vi "URL Equipos.vi"() -> ()   [LabVIEW 2018]
uses:
  <vilib>/RAFA Solutions/Harmony UI Controls Kit/Boolean/Blank Button - Green.ctl
  <vilib>/RAFA Solutions/Harmony UI Controls Kit/Boolean/Blank Button - Red.ctl
  <vilib>/RAFA Solutions/Harmony UI Controls Kit/String & Path/String Control.ctl
  <vilib>/RAFA Solutions/Harmony UI Controls Kit/Flat UI Design.lvlib
panel:
  out "NOMBRE 1":T1
  out "NOMBRE 2":T1
  out "NOMBRE 3":T1
  out "NOMBRE 4":T1
  out "NOMBRE 5":T1
  out "NOMBRE 6":T1
  out "IP 6":T1
  out "IP 5":T1
  out "IP 4":T1
  out "IP 3":T1
  out "IP 2":T1
  out "IP 1":T1
  in  "SALIR":T2
  in  "equipo 6":T3
  in  "equipo 5":T3
  in  "equipo 4":T3
  in  "equipo 3":T3
  in  "equipo 2":T3
  in  "equipo 1":T3
  # "URL EQUIPOS"
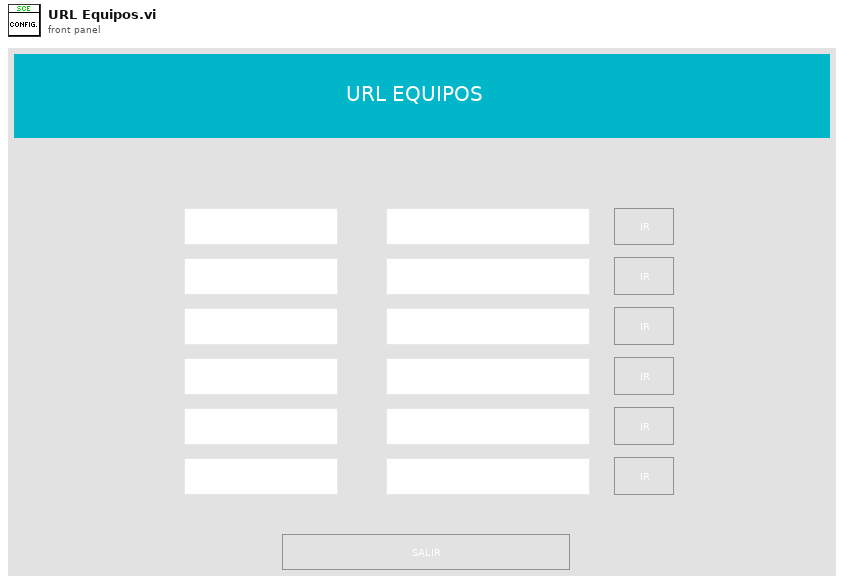
[diagram p1: front panel]
types:
  T1 = typedef "Flat UI Design.lvlib/String Control.ctl" = string
  T2 = typedef "Flat UI Design.lvlib/Blank Button - Red.ctl" = bool
  T3 = typedef "Flat UI Design.lvlib/Blank Button - Green.ctl" = bool
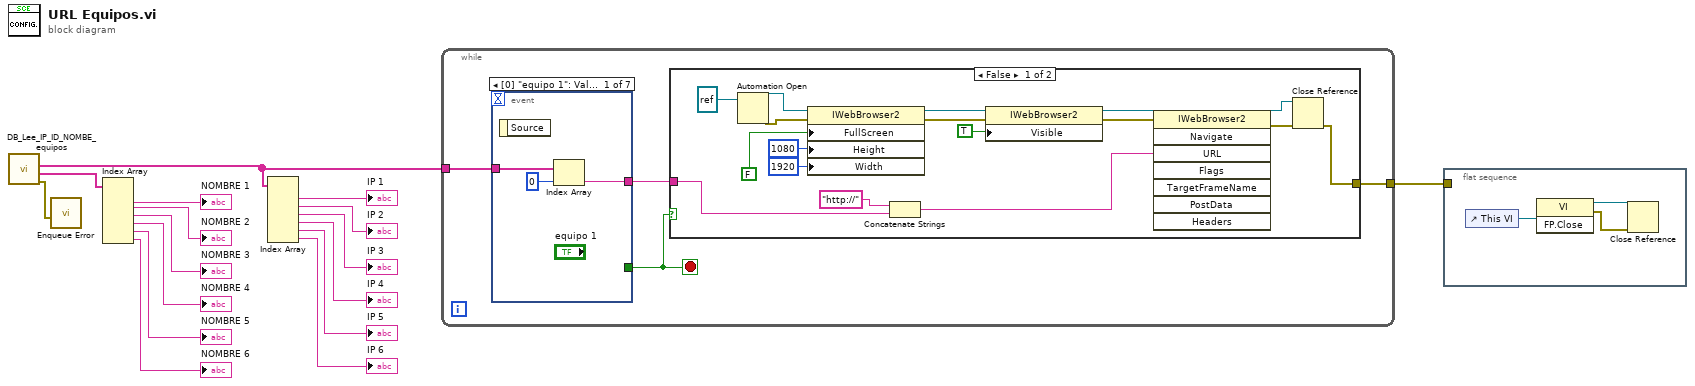
[diagram p0: block diagram]
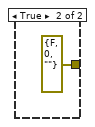
[diagram p2: hidden frame]
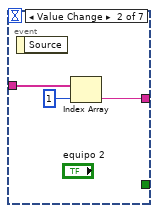
[diagram p3: hidden frame]
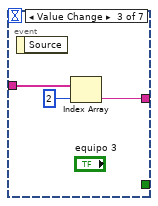
[diagram p4: hidden frame]
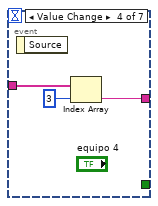
[diagram p5: hidden frame]
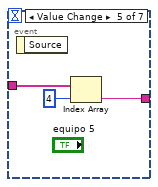
[diagram p6: hidden frame]
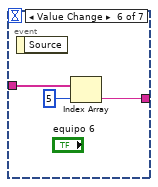
[diagram p7: hidden frame]
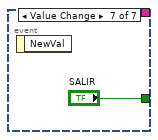
[diagram p8: hidden frame]
diagram:
  n1 = call "DB_Lee_IP_ID_NOMBE_equipos.vi"() -> ("error out"=w1:errorcluster, "NOMBRE_EQUIPOS"=w8:string[], "IP_EQUIPO"=w15:string[])  [unwired: 8 in, 1 out]
  n2 = call "Enqueue Error.vi"("error in"=w1) -> ()  [unwired: 9 in, 2 out]
  n3 = Index Array(array=w8) -> (element #1=→"NOMBRE 1":string, element #2=→"NOMBRE 2":string, element #3=→"NOMBRE 3":string, element #4=→"NOMBRE 4":string, element #5=→"NOMBRE 5":string, element #6=→"NOMBRE 6":string)  [unwired: 6 in]
  n4 = Index Array(array=w15) -> (element #1=→"IP 1":string, element #2=→"IP 2":string, element #3=→"IP 3":string, element #4=→"IP 4":string, element #5=→"IP 5":string, element #6=→"IP 6":string)  [unwired: 6 in]
  n5 = while {
    tunnel: [w19] -> w16
    tunnel: w15 -> [w18]
    stop <- w17 stop-if-true
    n6 = event shown="[0] \"equipo 1\": Value Change" {
      selector: _ -> [_ _ _ _ _ _ _]
      dyn-events: _ -> [_ _ _ _ _ _ _]
      timeout: _ -> [_ _ _ _ _ _ _]
      tunnel: w18 -> [w40 w43 w46 w49 w52 w55 _]
      tunnel: [w39 w42 w45 w48 w51 w54 _] -> w20
      tunnel: [_ _ _ _ _ _ "SALIR"] -> w17
      event Value Change {
        n7 = event-data() -> ()  [unwired: 1 in, 1 out]
        n8 = Index Array(array=w40, index=0 ("element")) -> (element=w39:string)
      }
      event Value Change {
        n9 = event-data() -> ()  [unwired: 1 in, 1 out]
        n10 = Index Array(array=w43, index=1 ("element")) -> (element=w42:string)
      }
      event Value Change {
        n11 = event-data() -> ()  [unwired: 1 in, 1 out]
        n12 = Index Array(array=w46, index=2 ("element")) -> (element=w45:string)
      }
      event Value Change {
        n13 = event-data() -> ()  [unwired: 1 in, 1 out]
        n14 = Index Array(array=w49, index=3 ("element")) -> (element=w48:string)
      }
      event Value Change {
        n15 = event-data() -> ()  [unwired: 1 in, 1 out]
        n16 = Index Array(array=w52, index=4 ("element")) -> (element=w51:string)
      }
      event Value Change {
        n17 = event-data() -> ()  [unwired: 1 in, 1 out]
        n18 = Index Array(array=w55, index=5 ("element")) -> (element=w54:string)
      }
      event Value Change {
        n19 = event-data() -> ()  [unwired: 1 in, 1 out]
      }
    }
    n20 = case shown="False" w17 {
      tunnel: w20 -> [w37 _]
      tunnel: [w36 errorcluster {"status"=FALSE, "code"=0, "source"=""} ("error out")] -> w19
      frame False {
        n21 = Automation Open(Automation Refnum=refnum<k7> refnum ("SHDocVw.IWebBrowser2")) -> (Automation Refnum=w35:refnum<k7>, error out=w34:errorcluster)  [unwired: 3 in]
        n22 = property class="IWebBrowser2"(reference=w35, error in=w34, "FullScreen"=FALSE, "Height"=1080, "Width"=1920) -> (reference out=w26:refnum<k7>, error out=w25:errorcluster)
        n23 = Concatenate Strings("http://" ("Enter a URL and run the VI"), w37) -> (w21:string)
        n24 = property class="IWebBrowser2"(reference=w26, error in=w25, "Visible"=TRUE) -> (reference out=w31:refnum<k7>, error out=w32:errorcluster)
        n25 = invoke class="IWebBrowser2" method="Navigate"(reference=w31, error in=w32, "URL"=w21) -> (reference out=w28:refnum<k7>, error out=w29:errorcluster)  [unwired: 5 in, 6 out]
        n26 = Close Reference(reference=w28, error in (no error)=w29) -> (error out=w36:errorcluster)
      }
      frame True {
      }
    }
  }
  n27 = flat-sequence {
    tunnel: w16 -> [_]
    frame #0 {
      n28 = control-ref of="This VI"() -> (w60:refnum<vi>)
      n29 = invoke class="VI" method="FP.Close"(reference=w60) -> (reference out=w59:refnum<vi>, error out=w58:errorcluster)  [unwired: 2 in, 1 out]
      n30 = Close Reference(reference=w59, error in (no error)=w58) -> ()  [unwired: 1 out]
    }
  }
